vi "Command-Line Get String Key.vi"(4 "string key":string) -> (0 "key found?":bool, 2 "string value":string)   [LabVIEW 2013]
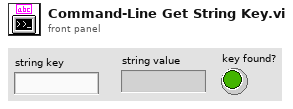
[diagram p1: front panel]
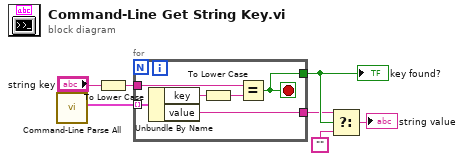
[diagram p0: block diagram]
diagram:
  n1 = call "Command-Line Parse All.vi"() -> ("string keys"=w7:cluster{"key":string, "value":string}[])  [unwired: 6 in, 5 out]
  n2 = To Lower Case(string="string key") -> (all lower case string=w6:string)
  n3 = for {
    tunnel: w7 -> [w13] mode=indexing
    tunnel: w6 -> [w10]
    tunnel: [w9] -> w4
    tunnel: [w8] -> w3
    stop <- w9 stop-if-true
    n4 = Unbundle By Name(w13) -> ("key"=w12:string, "value"=w8:string)
    n5 = To Lower Case(string=w12) -> (all lower case string=w11:string)
    n6 = Equal?(x=w10, y=w11) -> (x = y?=w9:bool)
  }
  "key found?" <- w4
  n7 = Select(t=w3, s=w4, f="") -> (s? t:f=→"string value":string)
